vi "user process.vi"(8 "error in":errorcluster, 11 "Parameters to process":T2) -> (0 "error out":errorcluster, 3 "Results from processing":T1)   [LabVIEW 2017, in "ExampleSequencer runtime.lvclass"]
uses:
  ExampleSequencer runtime.lvclass
  parameter user data.ctl
  result user data.ctl
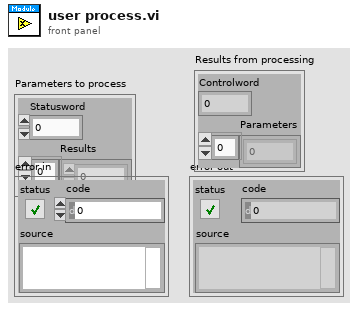
[diagram p1: front panel]
types:
  T1 = typedef "ExampleSequencer runtime.lvclass/result user data.ctl" = cluster{"Controlword":u16, "Parameters":dbl[]}
  T2 = typedef "ExampleSequencer runtime.lvclass/parameter user data.ctl" = cluster{"Statusword":u16, "Results":dbl[]}
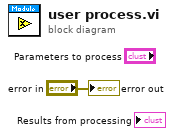
[diagram p0: block diagram]
diagram:
  "error out" <- "error in"
